vi "Write Key STR.vi"(7 "Section Name":string, 8 "error in":errorcluster, 9 "New Value":string, 10 "Key Name":string, 11 "Config Cluster in":T1) -> (0 "error out":errorcluster, 3 "Config Cluster out":T1)   [LabVIEW 2017]
uses:
  Config Cluster.ctl
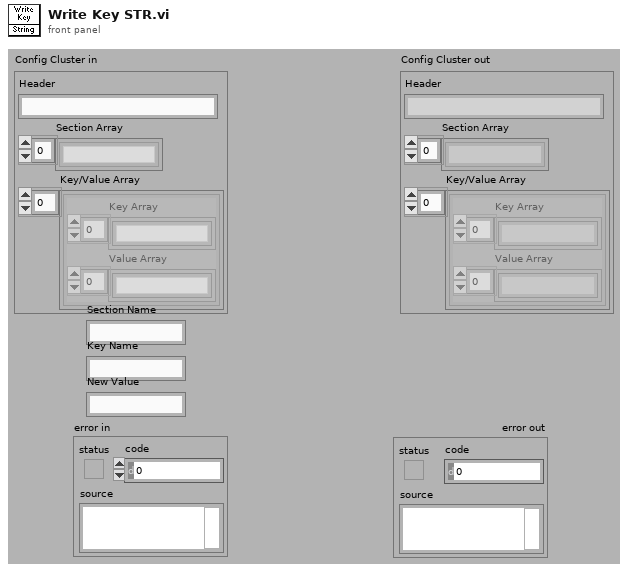
[diagram p1: front panel]
types:
  T1 = typedef "Config Cluster.ctl" = cluster{"Header":string, "Section Array":string[], "Key/Value Array":cluster{"Key Array":string[], "Value Array":string[]}[]}
  T2 = cluster{"Key Array":string[], "Value Array":string[]}[]
  T3 = cluster{"Key Array":string[], "Value Array":string[]}
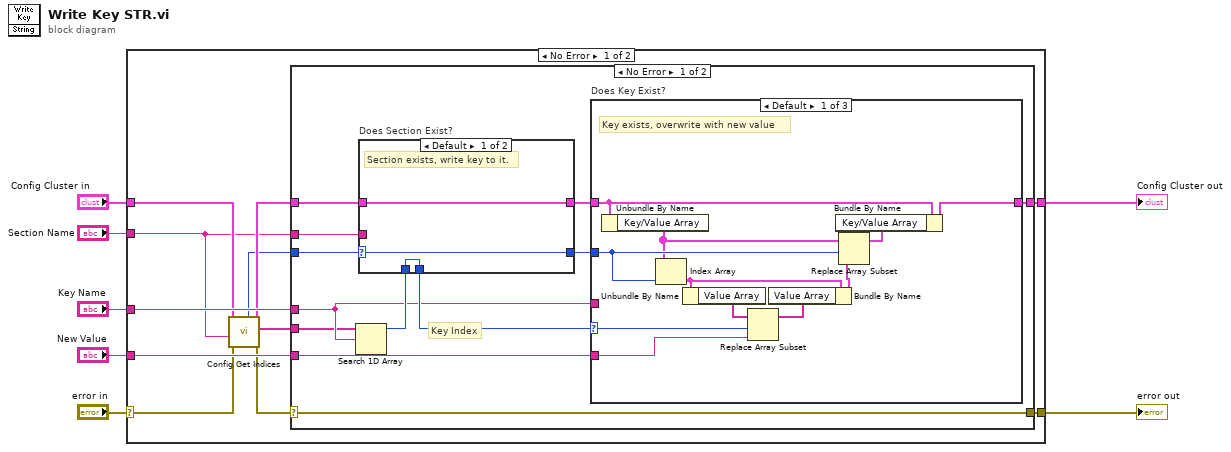
[diagram p0: block diagram]
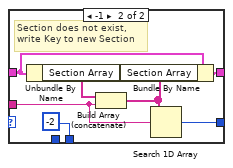
[diagram p2: hidden frame]
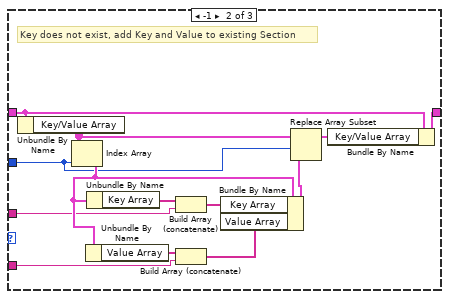
[diagram p3: hidden frame]
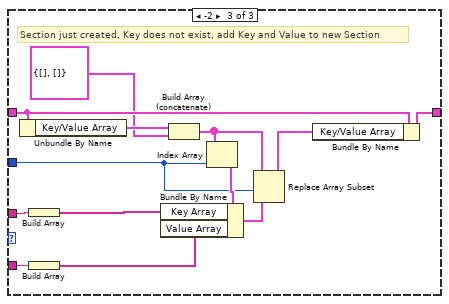
[diagram p4: hidden frame]
diagram:
  n1 = case shown="No Error" "error in" {
    selector: "error in" -> [w15 w80]
    tunnel: [w13 w80] -> w6
    tunnel: "Config Cluster in" -> [w14 w81]
    tunnel: [w11 w81] -> w4
    tunnel: "Section Name" -> [w9 _]
    tunnel: "Key Name" -> [w18 _]
    tunnel: "New Value" -> [w17 _]
    frame No Error {
      n2 = call "Config Get Indices.vi"("error in"=w15, "Section Name"=w9, "Config Cluster in"=w14) -> ("error out"=w16:errorcluster, "Key Array"=w10:string[], "Config Cluster out"=w12:T1, "Section Index"=w8:i32)  [unwired: 4 in, 1 out]
      n3 = case shown="No Error" w16 {
        selector: w16 -> [w23 w79]
        tunnel: w18 -> [w20 _]
        tunnel: w17 -> [w30 _]
        tunnel: w10 -> [w19 _]
        tunnel: [w23 w79] -> w13
        tunnel: w12 -> [w25 w78]
        tunnel: w8 -> [w28 _]
        tunnel: [w29 w78] -> w11
        tunnel: w9 -> [w26 _]
        frame No Error {
          # "Key Index"
          n4 = Search 1D Array(1D array=w19, element=w20) -> (index of element=w21:i32)  [unwired: 1 in]
          n5 = case "Does Section Exist?" shown="Default" w28 {
            selector: w28 -> [w33 _]
            tunnel: [w33 w37] -> w27
            tunnel: w26 -> [_ w35]
            tunnel: w25 -> [w32 w39]
            tunnel: [w32 w38] -> w24
            tunnel: w21 -> [w31 _]
            tunnel: [w31 -2] -> w22
            frame Default {
              # "Section exists, write key to it."
            }
            frame -1 {
              # "Section does not exist,\nwrite Key to new Section"
              n6 = Unbundle By Name(w39) -> ("Section Array"=w40:string[])
              n7 = Build Array (concatenate)(w40, w35) -> (w36:string[])
              n8 = Bundle By Name(cluster=w39, "Section Array"=w36) -> (w38:T1)
              n9 = Search 1D Array(1D array=w36, element=w35) -> (index of element=w37:i32)  [unwired: 1 in]
            }
          }
          n10 = case "Does Key Exist?" shown="Default" w22 {
            selector: w22 -> [w41 _ _]
            tunnel: w24 -> [w45 w64 w76]
            tunnel: w27 -> [w48 w57 w68]
            tunnel: w30 -> [w42 w61 w70]
            tunnel: [w44 w63 w77] -> w29
            tunnel: w20 -> [_ w52 w72]
            frame Default {
              # "Key exists, overwrite with new value"
              n11 = Unbundle By Name(w45) -> ("Key/Value Array"=w47:T2)
              n12 = Index Array(array=w47, index=w48) -> (element=w50:T3)
              n13 = Unbundle By Name(w50) -> ("Value Array"=w51:string[])
              n14 = Replace Array Subset(array=w51, new element=w42, index=w41) -> (w49:string[])
              n15 = Bundle By Name(cluster=w50, "Value Array"=w49) -> (w46:T3)
              n16 = Replace Array Subset(array=w47, new element=w46, index=w48) -> (w43:T2)
              n17 = Bundle By Name(cluster=w45, "Key/Value Array"=w43) -> (w44:T1)
            }
            frame -1 {
              # "Key does not exist, add Key and Value to existing Section"
              n18 = Unbundle By Name(w64) -> ("Key/Value Array"=w58:T2)
              n19 = Index Array(array=w58, index=w57) -> (element=w60:T3)
              n20 = Unbundle By Name(w60) -> ("Value Array"=w62:string[])
              n21 = Unbundle By Name(w60) -> ("Key Array"=w53:string[])
              n22 = Build Array (concatenate)(w53, w52) -> (w54:string[])
              n23 = Build Array (concatenate)(w62, w61) -> (w59:string[])
              n24 = Bundle By Name(cluster=w60, "Key Array"=w54, "Value Array"=w59) -> (w56:T3)
              n25 = Replace Array Subset(array=w58, new element=w56, index=w57) -> (w55:T2)
              n26 = Bundle By Name(cluster=w64, "Key/Value Array"=w55) -> (w63:T1)
            }
            frame -2 {
              # "Section just created, Key does not exist, add Key and Value to new Section"
              n27 = Unbundle By Name(w76) -> ("Key/Value Array"=w75:T2)
              n28 = Build Array(w72) -> (w71:string[])
              n29 = Build Array(w70) -> (w69:string[])
              n30 = Build Array (concatenate)(w75, cluster{string[], string[]} {[], []}) -> (w67:T2)
              n31 = Index Array(array=w67, index=w68) -> (element=w73:T3)
              n32 = Bundle By Name(cluster=w73, "Key Array"=w71, "Value Array"=w69) -> (w66:T3)
              n33 = Replace Array Subset(array=w67, new element=w66, index=w68) -> (w65:T2)
              n34 = Bundle By Name(cluster=w76, "Key/Value Array"=w65) -> (w77:T1)
            }
          }
        }
        frame Error {
        }
      }
    }
    frame Error {
    }
  }
  "error out" <- w6
  "Config Cluster out" <- w4
